vi "rsmxo_LV2015_Read_Waveform_Example.vi"() -> ()   [LabVIEW 2015]
uses:
  <instrlib>/Rohde&Schwarz MXO Oscilloscopes/Rohde&Schwarz MXO Oscilloscopes.lvlib
panel:
  in  "Record Length Limit":dbl=100000.0 caption="Record Length Limit (10000000)" format="%^.3e"
  in  "Time Scale":dbl=0.01 caption="Time Scale (20e-9)" format="%#.12p"
  in  "Coupling":i32(ring)=1 caption="Coupling (DC)" items=["DC", "DC Limit", "AC"]
  in  "Offset":dbl caption="Offset (0)" format="%#.12p"
  in  "Vertical Scale (per div)":dbl=0.1 caption="Vertical Scale (0.05)" format="%#.12p"
  out "Waveform Graph":T1(graph)={"X Start"=-0.05, "X Start"=1.0000000000000002e-08, "Waveform Data"=array[100000 elements]}
  in  "Maximum Wait Time":i32=10000 caption="Maximum Time (1000)"
  in  "Trigger Level":dbl=0.05 caption="Level (0)" format="%#.12p"
  in  "Trigger Slope":i32(ring)=2 caption="Slope (Either)" items=["Positive", "Negative", "Either"]
  in  "Trigger Mode":i32(ring) caption="Trigger Mode (Auto)" items=["Auto", "Normal", "Free Run"]
  in  "Channel":i32(ring)=1 caption="Channel (1)" items=["1"=1, "2"=2, "3"=3, "4"=4, "External"=5]
  in  "VISA resource name":refnum<visa-resource-name>="TCPIP::10.112.0.157::hislip0"
  in  "Reset":bool
  in  "ID Query":bool=TRUE
  # "Rohde & Schwarz RTM2000 Oscilloscope Read Waveform Example"
  # "Rohde & Schwarz RTx Oscilloscopes Series\nRead Waveform Example"
  # "Before running, change the VISA resource name to fit your device:\n- For LAN interface use TCPIP::<IP_Address>::INSTR e.g. TCPIP::10.64.0.178::INSTR\n- For USB interface use USB0::0x0AAD::<PID>::<SN>::INSTR e.g. USB0::0x0AAD::0x01D6::101457::INSTR\n- For GPIB interface use the GPIB::<Address>::INSTR e.g. GPIB::28::INSTR"
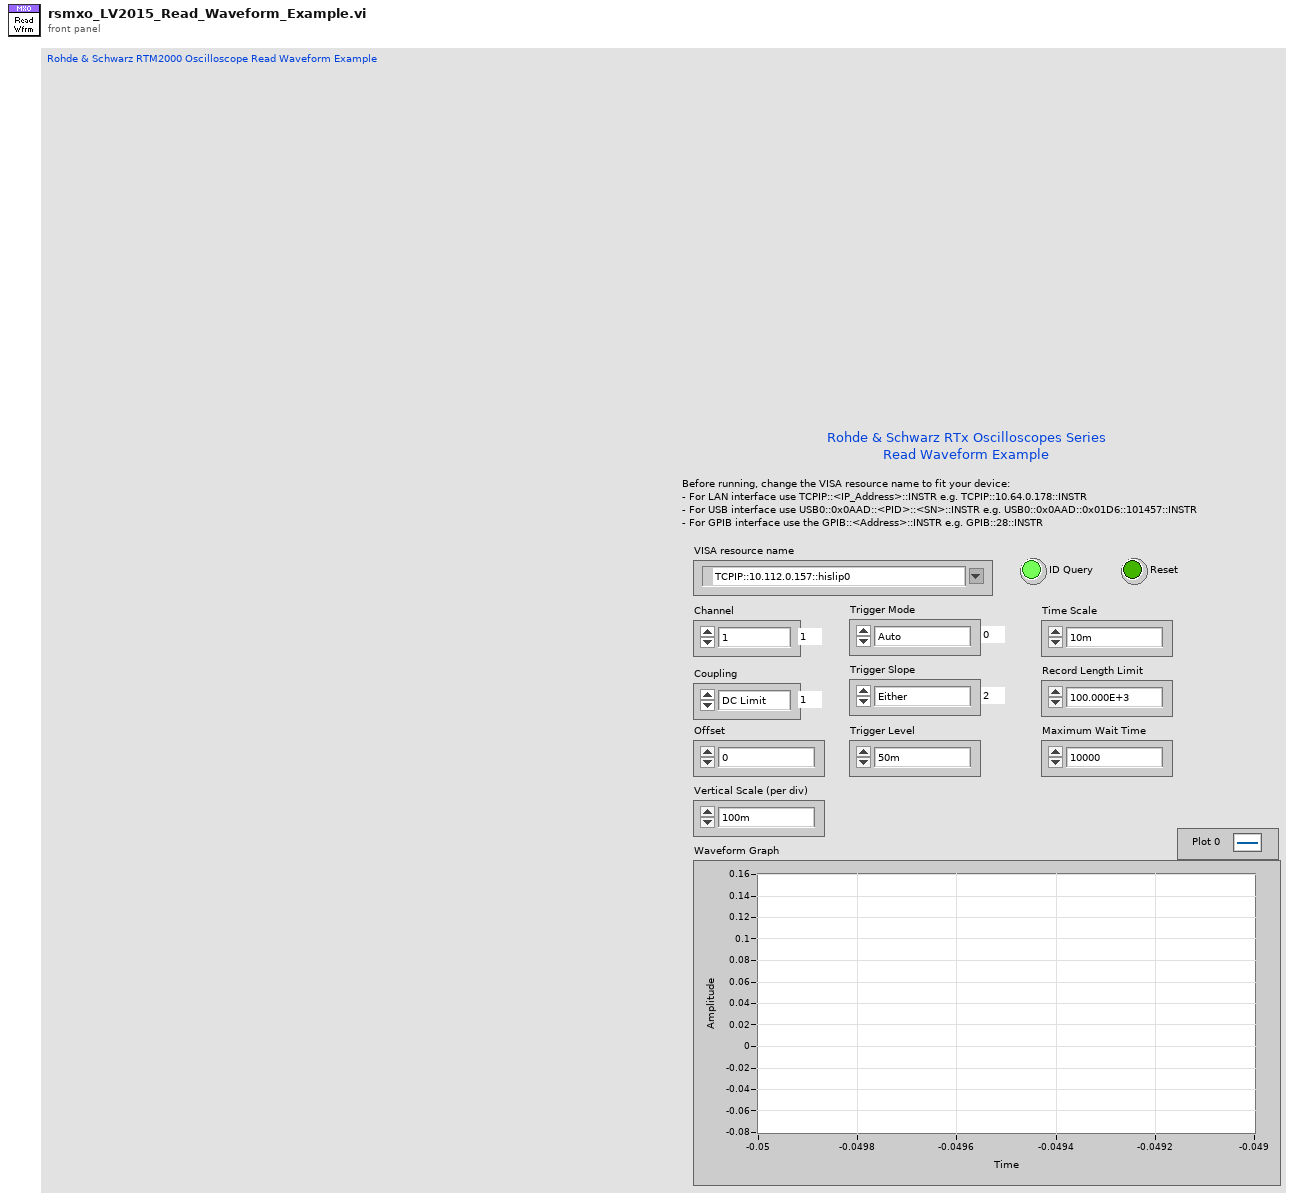
[diagram p1: front panel]
types:
  T1 = cluster{"X Start":dbl, "X Start":dbl, "Waveform Data":dbl[]}
  T2 = cluster{"X Start":dbl, dbl, "Waveform Data":dbl[]}
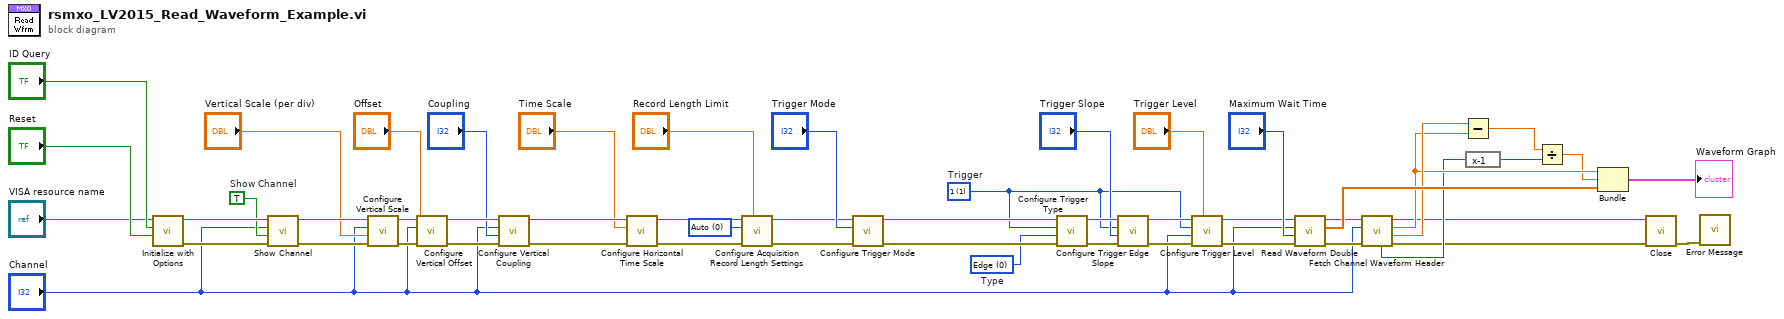
[diagram p0: block diagram]
diagram:
  w9 = 0 items=["Auto", "Manual"] ("Mode (Auto)")
  w20 = TRUE  # Show Channel
  w44 = 0 items=["Edge", "Glitch", "Width", "Runt", "Window", "Timeout", "Interval", "Slewrate", "Sethold", "State", "Pattern", "Analog Edge"]  # Type
  w38 = 1 items=["1"=1, "2"=2, "3"=3]  # Trigger
  n1 = call <instrlib>:"Initialize with Options.vi"("Reset (T: Reset)"="Reset", "ID Query (T: Check)"="ID Query", "VISA resource name"="VISA resource name") -> ("error out"=w28:errorcluster, "VISA resource name out"=w27:refnum<visa-resource-name>)  [unwired: 7 in]
  n2 = call <instrlib>:"Show Channel.vi"("error in (no error)"=w28, "Show Channel (Off)"=w20, "Channel (1)"="Channel", "VISA resource name"=w27) -> ("error out"=w26:errorcluster, "VISA resource name out"=w25:refnum<visa-resource-name>)  [unwired: 6 in]
  n3 = call <instrlib>:"Configure Vertical Scale.vi"("error in (no error)"=w26, "Vertical Scale (0.05)"="Vertical Scale (per div)", "Channel (1)"="Channel", "VISA resource name"=w25) -> ("error out"=w24:errorcluster, "VISA resource name out"=w23:refnum<visa-resource-name>)  [unwired: 6 in]
  n4 = call <instrlib>:"Configure Vertical Offset.vi"("error in (no error)"=w24, "Offset (0)"="Offset", "Channel (1)"="Channel", "VISA resource name"=w23) -> ("error out"=w22:errorcluster, "VISA resource name out"=w21:refnum<visa-resource-name>)  [unwired: 6 in]
  n5 = call <instrlib>:"Configure Vertical Coupling.vi"("error in (no error)"=w22, "Coupling (DC)"="Coupling", "Channel (1)"="Channel", "VISA resource name"=w21) -> ("error out"=w16:errorcluster, "VISA resource name out"=w15:refnum<visa-resource-name>)  [unwired: 6 in]
  n6 = call <instrlib>:"Configure Horizontal Time Scale.vi"("error in (no error)"=w16, "Time Scale (20e-9)"="Time Scale", "VISA resource name"=w15) -> ("error out"=w13:errorcluster, "VISA resource name out"=w12:refnum<visa-resource-name>)  [unwired: 7 in]
  n7 = call <instrlib>:"Configure Acquisition Record Length Settings.vi"("Record Length Limit (10000000)"="Record Length Limit", "error in (no error)"=w13, "Mode (Auto)"=w9, "VISA resource name"=w12) -> ("error out"=w11:errorcluster, "VISA resource name out"=w10:refnum<visa-resource-name>)  [unwired: 6 in]
  n8 = call <instrlib>:"Configure Trigger Mode.vi"("error in (no error)"=w11, "Trigger Mode (Auto)"="Trigger Mode", "VISA resource name"=w10) -> ("error out"=w47:errorcluster, "VISA resource name out"=w46:refnum<visa-resource-name>)  [unwired: 7 in]
  n9 = call <instrlib>:"Configure Trigger Type.vi"("error in (no error)"=w47, "Type (Edge)"=w44, "Trigger (1)"=w38, "VISA resource name"=w46) -> ("error out"=w43:errorcluster, "VISA resource name out"=w42:refnum<visa-resource-name>)  [unwired: 6 in]
  n10 = call <instrlib>:"Configure Trigger Edge Slope.vi"("error in (no error)"=w43, "Slope (Either)"="Trigger Slope", "Trigger (1)"=w38, "VISA resource name"=w42) -> ("error out"=w41:errorcluster, "VISA resource name out"=w40:refnum<visa-resource-name>)  [unwired: 6 in]
  n11 = call <instrlib>:"Configure Trigger Level.vi"("Level (0)"="Trigger Level", "error in (no error)"=w41, "Channel (1)"="Channel", "Trigger (1)"=w38, "VISA resource name"=w40) -> ("error out"=w7:errorcluster, "VISA resource name out"=w6:refnum<visa-resource-name>)  [unwired: 5 in]
  n12 = call <instrlib>:"Read Waveform Double.vi"("error in (no error)"=w7, "Timeout in ms (0 - current OPC timeout)"="Maximum Wait Time", "Source (Channel 1)"="Channel", "VISA resource name"=w6) -> ("error out"=w5:errorcluster, "Waveform Data"=w49:dbl[], "VISA resource name out"=w4:refnum<visa-resource-name>)  [unwired: 5 in]
  n13 = call <instrlib>:"Fetch Channel Waveform Header.vi"("error in (no error)"=w5, "Channel (1)"="Channel", "VISA resource name"=w4) -> ("error out"=w2:errorcluster, "X Stop"=w34:dbl, "X Start"=w33:dbl, "VISA resource name out"=w1:refnum<visa-resource-name>, "Record Length"=w31:i32)  [unwired: 3 in, 1 out]
  n14 = Subtract(x=w34, y=w33) -> (x-y=w32:dbl)
  n15 = expression code="x-1"(w31) -> (w30:i32)
  n16 = Divide(x=w32, y=w30) -> (x/y=w29:dbl)
  n17 = Bundle("X Start"=w33, w29, "Waveform Data"=w49) -> (→"Waveform Graph":T2)  [unwired: 1 in]
  n18 = call <instrlib>:"Close.vi"("error in (no error)"=w2, "VISA resource name"=w1) -> ("error out"=w48:errorcluster)  [unwired: 9 in]
  n19 = call <instrlib>:"Error Message.vi"("error in (no error)"=w48) -> ()  [unwired: 10 in, 5 out]
